vi "New.vi"(6 "Timeout ms (25000)":i32=25000, 7 "Max size (548)":i32=548, 8 "Error In":errorcluster, 11 "Port (61557)":u16=61557) -> (0 "Error Out":errorcluster, 3 "Receiver Ref.":refnum<class "Receiver.lvclass">)   [LabVIEW 2020, in "RemoteVariables.lvlib" / "Receiver.lvclass"]
uses:
  Receiver.lvclass
  Receiver.lvclass/Receiver.ctl
  UDP/UDP.lvclass
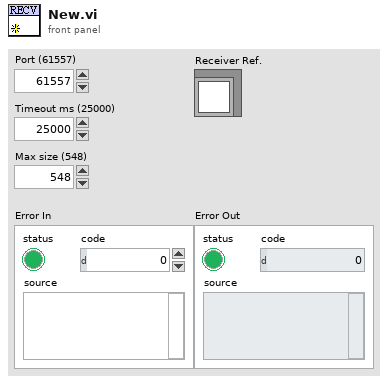
[diagram p1: front panel]
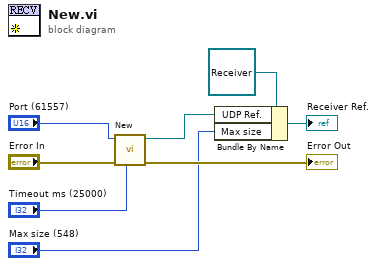
[diagram p0: block diagram]
diagram:
  n1 = call "New.vi"("Timeout ms (25000)"="Timeout ms (25000)", "Error In"="Error In", "Port (61557)"="Port (61557)") -> ("Error Out"=→"Error Out":errorcluster, "UDP Ref."=w5:refnum<class "UDP.lvclass">)  [unwired: 7 in]
  n2 = Bundle By Name(cluster=refnum<class "Receiver.lvclass"> refnum ("RemoteVariables.lvlib:Receiver.lvclass"), "UDP Ref."=w5, "Max size"="Max size (548)") -> (→"Receiver Ref.":refnum<class "Receiver.lvclass">)
